vi "SharedVariable.Read.vi"(8 "error in":errorcluster, 9 "default value":string, 10 "variable":string) -> (0 "error out":errorcluster, 1 "found":bool, 2 "value":string)   [LabVIEW 2019, in "Tools.lvlib"]
uses:
  Tools.lvlib
  ProjectPaths.vi
  <vilib>/Utility/config.llb/Read Key (String).vi
  <vilib>/Utility/config.llb/NI_LVConfig.lvlib
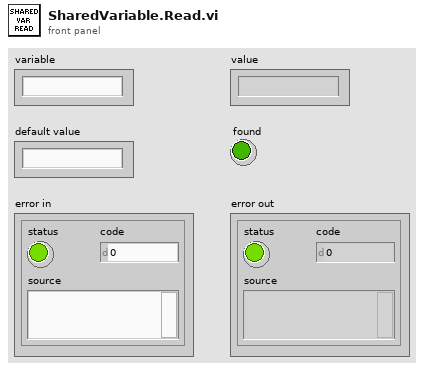
[diagram p1: front panel]
types:
  T1 = typedef "NI_LVConfig.lvlib/Config Data RefNum.ctl" = refnum<k1>
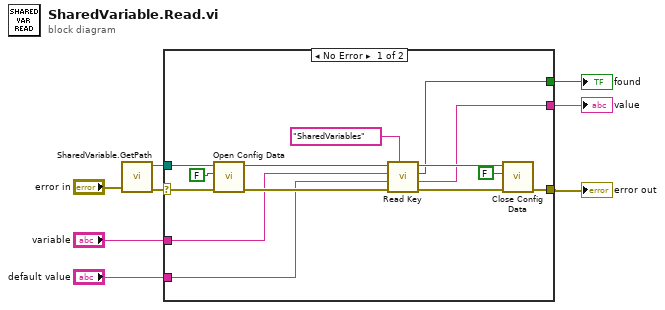
[diagram p0: block diagram]
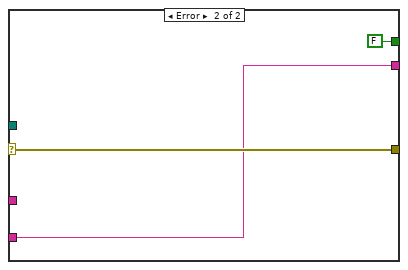
[diagram p2: hidden frame]
diagram:
  n1 = call "SharedVariable.GetPath.vi"("error in (no error)"="error in") -> ("error out"=w1:errorcluster, "Shared Variables path"=w3:path)  [unwired: 9 in]
  n2 = case shown="No Error" w1 {
    selector: w1 -> [w21 w25]
    tunnel: w3 -> [w20 _]
    tunnel: "variable" -> [w11 _]
    tunnel: [w13 FALSE ("found?")] -> w7
    tunnel: [w14 w25] -> w8
    tunnel: [w12 w23] -> w4
    tunnel: "default value" -> [w9 w23]
    frame No Error {
      n3 = call <vilib>:"Open Config Data.vi"("error in (no error)"=w21, "create file if necessary (T)"=FALSE, "configuration file path"=w20) -> ("error out"=w19:errorcluster, "refnum"=w18:T1)  [unwired: 6 in, 1 out]
      n4 = call-poly <vilib>:"Read Key.vi"("section"="SharedVariables", "error in (no error)"=w19, "default value"=w9, "key"=w11, "refnum"=w18) -> ("error out"=w17:errorcluster, "value"=w12:string, "found?"=w13:bool, "refnum out"=w16:T1)  [unwired: 3 in]
      n5 = call <vilib>:"Close Config Data.vi"("error in (no error)"=w17, "write file if changed (T)"=FALSE, "refnum"=w16) -> ("error out"=w14:errorcluster)  [unwired: 7 in, 1 out]
    }
    frame Error {
    }
  }
  "error out" <- w8
  "found" <- w7
  "value" <- w4
